vi "T7 Checksum KAG.vi"(11 "Array":u8[](array[numeric])=[139, 242, 0, 160, 247, 0] format="%.0x") -> (0 "Checksum Error":bool, 1 "Array Output":u8[](array[numeric])=[139, 242, 0, 160, 247, 0] format="%.0x", 2 "Calculated Checksum8":u8 format="%.0x", 3 "Input Checksum8":u8 format="%.0x", 4 "Calculated Checksum16 MSB":u8 format="%.0x", 5 "Input Checksum16 MSB":u8 format="%.0x", 6 "Calculated Checksum16 LSB":u8 format="%.0x", 7 "Input Checksum16 LSB":u8 format="%.0x")   [LabVIEW 2015]
panel:
  # "Checksum8"
  # "Checksum16 MSB"
  # "Checksum16 LSB"
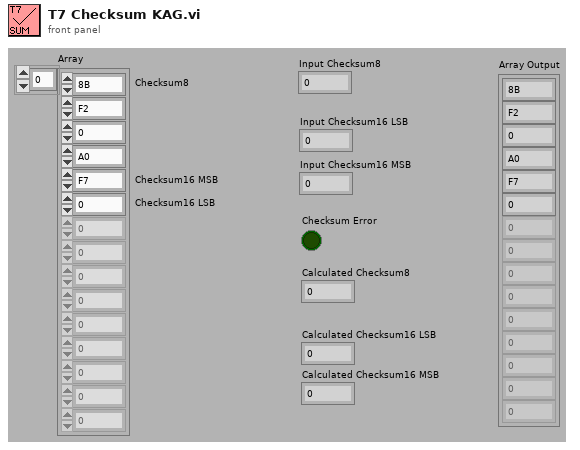
[diagram p1: front panel]
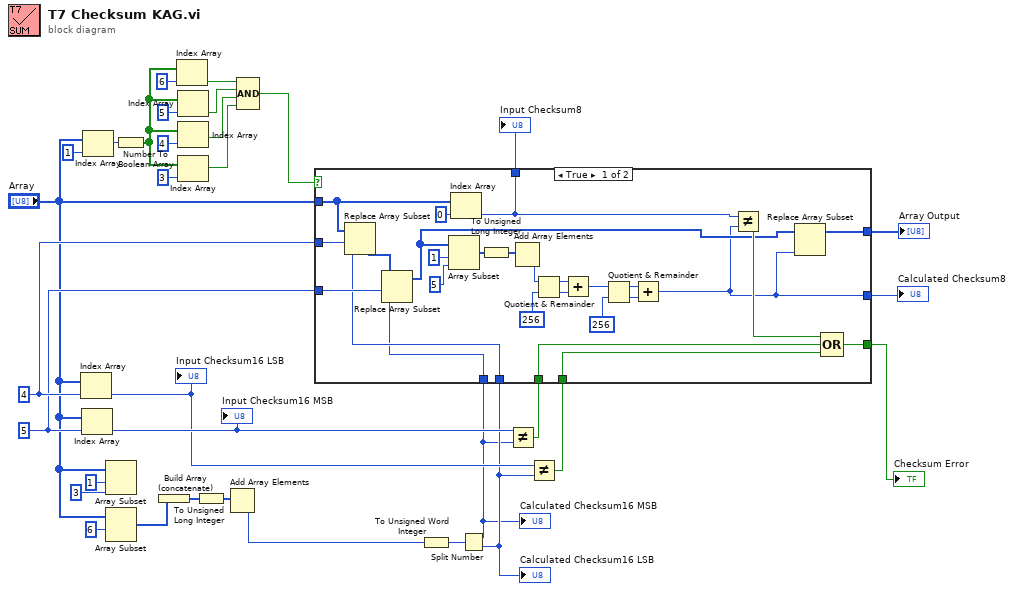
[diagram p0: block diagram]
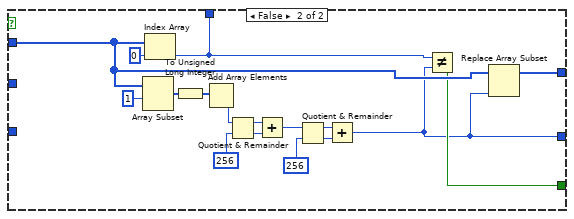
[diagram p2: hidden frame]
diagram:
  w22 = 5 ("Index")
  w23 = 4 ("Index")
  n1 = Index Array(array="Array", index=w23) -> (element=w27:u8)
  "Input Checksum16 LSB" <- w27
  n2 = Index Array(array="Array", index=w22) -> (element=w28:u8)
  "Input Checksum16 MSB" <- w28
  n3 = Index Array(array="Array", index=1 ("Index")) -> (element=w13:u8)
  n4 = Array Subset(array="Array", index=1 ("Array Index"), length=3 ("Array Length")) -> ()  [unwired: 1 out]
  n5 = Array Subset(array="Array", index=6 ("Array Index")) -> (w1:u8[])  [unwired: 1 in]
  n6 = Number To Boolean Array(number=w13) -> (Boolean array=w8:bool[])
  n7 = Build Array (concatenate)(w1) -> (w29:u8[])
  n8 = Index Array(array=w8, index=6 ("Index")) -> (element=w7:bool)
  n9 = Index Array(array=w8, index=5 ("Index")) -> (element=w6:bool)
  n10 = Index Array(array=w8, index=4 ("Index")) -> (element=w5:bool)
  n11 = Index Array(array=w8, index=3 ("Index")) -> (element=w4:bool)
  n12 = To Unsigned Long Integer(number=w29) -> (unsigned 32bit integer=w30:u32[])
  n13 = Add Array Elements(numeric array=w30) -> (sum=w2:u32)
  n14 = Compound Arithmetic op=AND(w7, w6, w5, w4) -> (w3:bool)
  n15 = To Unsigned Word Integer(number=w2) -> (unsigned 16bit integer=w16:u16)
  n16 = Split Number(x=w16) -> (hi(x)=w20:u8, lo(x)=w21:u8)
  "Calculated Checksum16 MSB" <- w20
  "Calculated Checksum16 LSB" <- w21
  n17 = Not Equal?(x=w28, y=w20) -> (x != y?=w26:bool)
  n18 = Not Equal?(x=w27, y=w21) -> (x != y?=w25:bool)
  n19 = case shown="True" w3 {
    tunnel: w26 -> [w52 _]
    tunnel: w25 -> [w51 _]
    tunnel: [w50 w66] -> w24
    tunnel: "Array" -> [w48 w67]
    tunnel: w23 -> [w47 _]
    tunnel: w22 -> [w46 _]
    tunnel: w21 -> [w45 _]
    tunnel: w20 -> [w44 _]
    tunnel: [w43 w69] -> w19
    tunnel: [w41 w68] -> w18
    tunnel: [w34 w61] -> w17
    frame True {
      n20 = Replace Array Subset(array=w48, new element=w45, index=w47) -> (w49:u8[])
      n21 = Replace Array Subset(array=w49, new element=w44, index=w46) -> (w40:u8[])
      n22 = Array Subset(array=w40, index=1 ("Array Index"), length=5 ("Array Length")) -> (w54:u8[])
      n23 = Index Array(array=w48, index=0 ("Index")) -> (element=w41:u8)
      n24 = To Unsigned Long Integer(number=w54) -> (unsigned 32bit integer=w53:u32[])
      n25 = Add Array Elements(numeric array=w53) -> (sum=w56:u32)
      n26 = Quotient & Remainder(x=w56, y=u16 256) -> (x-y*floor(x/y)=w59:u32, floor(x/y)=w58:u32)
      n27 = Add(x=w59, y=w58) -> (x+y=w35:u32)
      n28 = Quotient & Remainder(x=w35, y=u16 256) -> (x-y*floor(x/y)=w37:u32, floor(x/y)=w36:u32)
      n29 = Add(x=w37, y=w36) -> (x+y=w34:u32)
      n30 = Not Equal?(x=w41, y=w34) -> (x != y?=w42:bool)
      n31 = Replace Array Subset(array=w40, new element=w34) -> (w43:u8[])  [unwired: 1 in]
      n32 = Compound Arithmetic op=OR(w42, w52, w51) -> (w50:bool)
    }
    frame False {
      n33 = Array Subset(array=w67, index=1 ("Array Index")) -> (w71:u8[])  [unwired: 1 in]
      n34 = Index Array(array=w67, index=0 ("Index")) -> (element=w68:u8)
      n35 = To Unsigned Long Integer(number=w71) -> (unsigned 32bit integer=w70:u32[])
      n36 = Add Array Elements(numeric array=w70) -> (sum=w73:u32)
      n37 = Quotient & Remainder(x=w73, y=u16 256) -> (x-y*floor(x/y)=w76:u32, floor(x/y)=w75:u32)
      n38 = Add(x=w76, y=w75) -> (x+y=w62:u32)
      n39 = Quotient & Remainder(x=w62, y=u16 256) -> (x-y*floor(x/y)=w64:u32, floor(x/y)=w63:u32)
      n40 = Add(x=w64, y=w63) -> (x+y=w61:u32)
      n41 = Not Equal?(x=w68, y=w61) -> (x != y?=w66:bool)
      n42 = Replace Array Subset(array=w67, new element=w61) -> (w69:u8[])  [unwired: 1 in]
    }
  }
  "Calculated Checksum8" <- w17
  "Input Checksum8" <- w18
  "Checksum Error" <- w24
  "Array Output" <- w19
